vi "UpdateVI.vi"(8 "error in (no error)":errorcluster, 10 "Controls":path, 11 "VIToUpdate":path) -> (0 "error out":errorcluster)   [LabVIEW 2015]
uses:
  <vilib>/Utility/traverseref.llb/TRef TravTarget.ctl
  <vilib>/Utility/traverseref.llb/VI Scripting - Traverse.lvlib
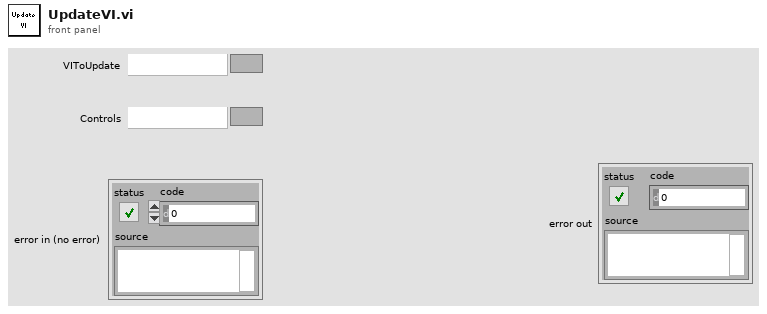
[diagram p1: front panel]
types:
  T1 = typedef "TRef TravTarget.ctl" = enum16{"FP", "BD", "Other"}
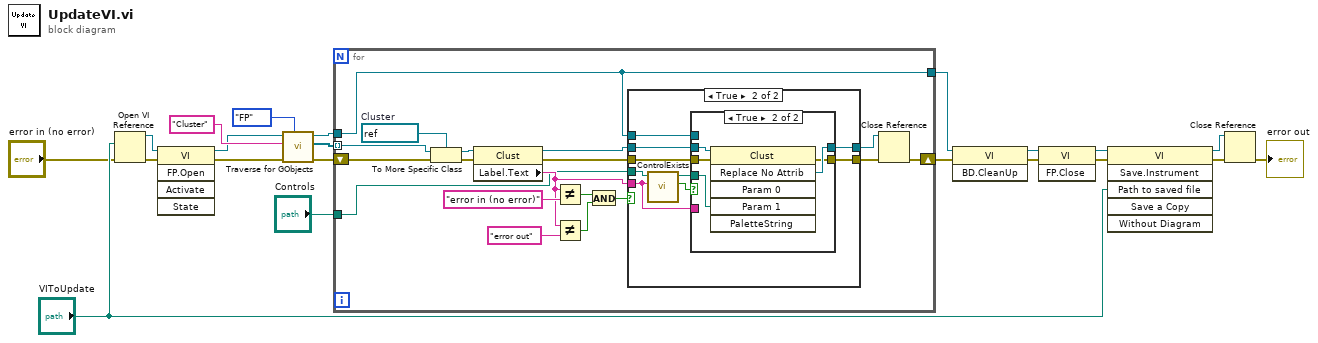
[diagram p0: block diagram]
diagram:
  n1 = Open VI Reference(vi path="VIToUpdate", error in (no error)="error in (no error)") -> (vi reference=w15:refnum<vi>, error out=w9:errorcluster)  [unwired: 4 in]
  n2 = invoke class="VI" method="FP.Open"(reference=w15, error in=w9) -> (reference out=w10:refnum<vi>, error out=w8:errorcluster)  [unwired: 3 in, 3 out]
  n3 = call <vilib>:"Traverse for GObjects.vi"("Traverse Target"=TRef_TravTarget."FP", "error in (no error)"=w8, "Class Name"="Cluster", "VI Refnum"=w10) -> ("error out"=w17:errorcluster, "References"=w19:refnum<vi>[], "dup VI Refnum"=w18:refnum<vi>)  [unwired: 4 in, 1 out]
  n4 = for {
    tunnel: w19 -> [w37] mode=indexing
    tunnel: w18 -> [w22]
    shift-right: [w25] -> w14
    shift-left: w17 -> [w38]
    tunnel: "Controls" -> [w23]
    tunnel: [w22] -> w13
    w39 = refnum<vi> refnum  # Cluster
    n5 = To More Specific Class(target class=w39, reference=w37, error in=w38) -> (specific class reference=w36:refnum<vi>, error out=w35:errorcluster)
    n6 = property class="Clust"(reference=w36, error in=w35) -> (reference out=w27:refnum<vi>, error out=w29:errorcluster, "Label.Text"=w28:string)
    n7 = Not Equal?(x=w28, y="error in (no error)") -> (x != y?=w33:bool)
    n8 = Not Equal?(x=w28, y="error out") -> (x != y?=w34:bool)
    n9 = And(x=w33, y=w34) -> (x .and. y?=w30:bool)
    n10 = case shown="True" w30 {
      tunnel: w29 -> [w40 w50]
      tunnel: w28 -> [_ w45]
      tunnel: w27 -> [w41 w49]
      tunnel: [w40 w48] -> w26
      tunnel: [w41 w47] -> w24
      tunnel: w23 -> [_ w46]
      tunnel: w22 -> [_ w42]
      frame False {
      }
      frame True {
        n11 = call "ControlExists.vi"("ControlName"=w45, "ControlsPath"=w46) -> ("Boolean"=w44:bool, "ControlPath"=w43:path)  [unwired: 8 in]
        n12 = case shown="True" w44 {
          tunnel: w50 -> [w52 w55]
          tunnel: w49 -> [w51 w56]
          tunnel: [w52 w53] -> w48
          tunnel: [w51 w54] -> w47
          tunnel: w45 -> [_ _]
          tunnel: w43 -> [_ w57]
          tunnel: w42 -> [_ _]
          frame False {
          }
          frame True {
            n13 = invoke class="Clust" method="Replace No Attrib"(reference=w56, error in=w55, "Param 1"=w57) -> (error out=w53:errorcluster, "RepNoAttrib"=w54:refnum<vi>)  [unwired: 3 in, 4 out]
          }
        }
      }
    }
    n14 = Close Reference(reference=w24, error in (no error)=w26) -> (error out=w25:errorcluster)
  }
  n15 = invoke class="VI" method="BD.CleanUp"(reference=w13, error in=w14) -> (reference out=w12:refnum<vi>, error out=w11:errorcluster)  [unwired: 1 in, 1 out]
  n16 = invoke class="VI" method="FP.Close"(reference=w12, error in=w11) -> (reference out=w7:refnum<vi>, error out=w6:errorcluster)  [unwired: 1 in, 1 out]
  n17 = invoke class="VI" method="Save.Instrument"(reference=w7, error in=w6, "Path to saved file"="VIToUpdate") -> (reference out=w4:refnum<vi>, error out=w3:errorcluster)  [unwired: 3 in, 4 out]
  n18 = Close Reference(reference=w4, error in (no error)=w3) -> (error out=→"error out":errorcluster)
